vi "Add Default Enum.vi"(6 "Hdr Name":T1, 8 "error in (no error)":errorcluster, 9 "Enum Values":u16[](array[numeric]), 11 "Strain in":refnum<class "Strain.lvclass">) -> (0 "error out":errorcluster, 3 "Strain out":refnum<class "Strain.lvclass">)   [LabVIEW 2018, in "Measurement Channels.lvlib" / "Strain.lvclass"]
uses:
  Strain.lvclass
  Common/Controls/HeaderNames.ctl
  Strain.lvclass/Strain.ctl
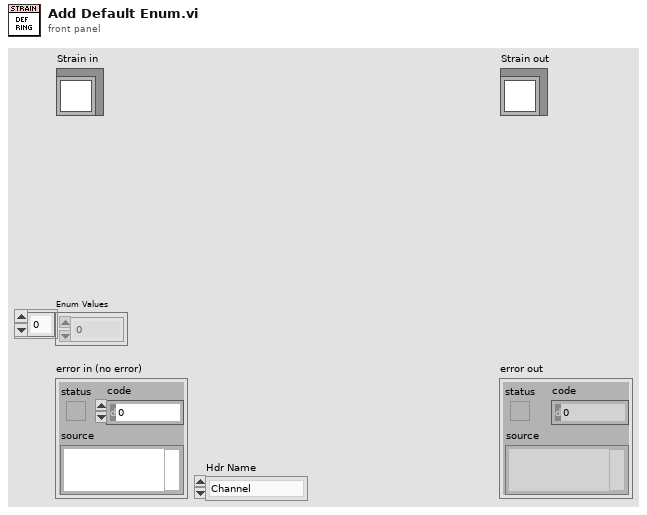
[diagram p1: front panel]
types:
  T1 = typedef "HeaderNames.ctl" = enum16{"Channel", "Device", "Spacer", "Description", "MB", "Range", "Terminal", "Coupling", "Thresh (V)", "Pulse/Rev", "Slope", "Min EU", "Min RPM", "mV/EU", "Iex", "Temp Units", "Type", "CJC Src", "CJC Val", "Ro", "Wire Cfg", "Strain Mode", "Vex", "Bridge Type", "GF", "Gauge Res", "Poisson", "Lead Res", "Init Strain", "GAF", "Scale", "Offset", "Unit (EU)", "dB?", "dB Ref", "Cal Mag", "Cal Units", "Max Temp", "Min Temp", "Max Strain", "Min Strain"}
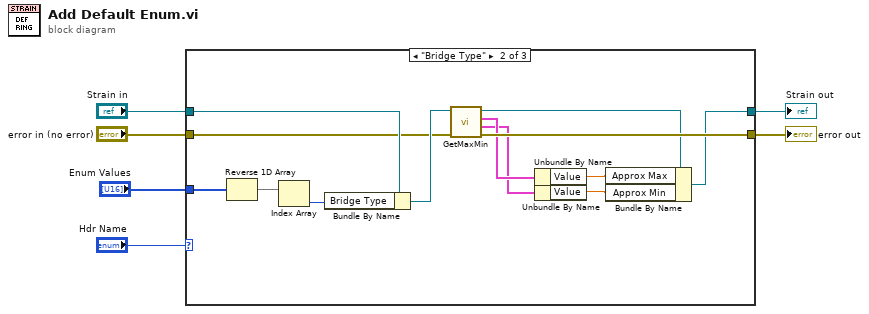
[diagram p0: block diagram]
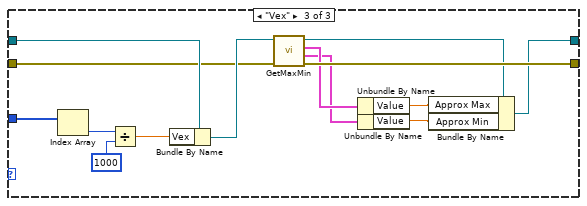
[diagram p3: hidden frame]
diagram:
  n1 = case shown="\"Bridge Type\"" "Hdr Name" {
    tunnel: "Strain in" -> [w8 w21 w35]
    tunnel: "error in (no error)" -> [w7 w19 w33]
    tunnel: [w8 w13 w30] -> w3
    tunnel: [w7 w18 w32] -> w2
    tunnel: "Enum Values" -> [_ w15 w23]
    frame Default {
    }
    frame "Bridge Type" {
      n2 = Reverse 1D Array(array=w15) -> (reversed array=w17:u16[])
      n3 = Index Array(array=w17) -> (element=w16:u16)  [unwired: 1 in]
      n4 = Bundle By Name(cluster=w21, "Bridge Type"=w16) -> (w20:refnum<class "Strain.lvclass">)
      n5 = call-dynamic "GetMaxMin.vi"("error in (no error)"=w19, "Strain in"=w20) -> ("error out"=w18:errorcluster, "Min"=w9:cluster{"Value":dbl, "Text":string}, "Max"=w12:cluster{"Value":dbl, "Text":string}, "Strain out"=w14:refnum<class "Strain.lvclass">)  [unwired: 6 in]
      n6 = Unbundle By Name(w12) -> ("Value"=w11:dbl)
      n7 = Unbundle By Name(w9) -> ("Value"=w10:dbl)
      n8 = Bundle By Name(cluster=w14, "Approx Max"=w11, "Approx Min"=w10) -> (w13:refnum<class "Strain.lvclass">)
    }
    frame "Vex" {
      n9 = Index Array(array=w23) -> (element=w25:u16)  [unwired: 1 in]
      n10 = Divide(x=w25, y=1000) -> (x/y=w22:dbl)
      n11 = Bundle By Name(cluster=w35, "Vex"=w22) -> (w34:refnum<class "Strain.lvclass">)
      n12 = call-dynamic "GetMaxMin.vi"("error in (no error)"=w33, "Strain in"=w34) -> ("error out"=w32:errorcluster, "Min"=w26:cluster{"Value":dbl, "Text":string}, "Max"=w29:cluster{"Value":dbl, "Text":string}, "Strain out"=w31:refnum<class "Strain.lvclass">)  [unwired: 6 in]
      n13 = Unbundle By Name(w29) -> ("Value"=w28:dbl)
      n14 = Unbundle By Name(w26) -> ("Value"=w27:dbl)
      n15 = Bundle By Name(cluster=w31, "Approx Max"=w28, "Approx Min"=w27) -> (w30:refnum<class "Strain.lvclass">)
    }
  }
  "error out" <- w2
  "Strain out" <- w3
